vi "手动静音-网络版.vi"(9 "引用-通信单元-探头属性引用[]":refnum<vi>, 10 "引用-通信单元-改动项引用[]":refnum<vi>, 11 "引用-测量状态":refnum<vi>) -> ()   [LabVIEW 2017]
panel:
  in  "列表框":i32(listbox)
  out "映射-改动项引用[]":refnum<vi>[](array[refnum])
  in  "事件-选中行":refnum<user-event>
  in  "选中行":i32[](array[numeric])
  out "项数":i32
  out "信号-刷新列表":bool=TRUE
  in  "上翻":bool
  in  "全部静音":bool
  in  "下翻":bool
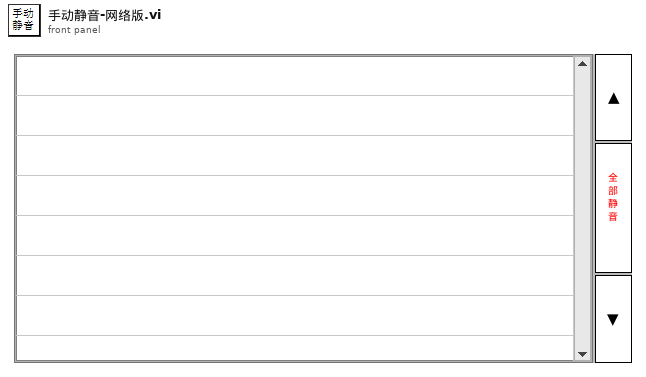
[diagram p1: front panel]
types:
  T1 = typedef "测量状态.ctl" = enum16{"正常", "一级报警", "二级报警", "累积报警", "有掉线"}
  T2 = typedef "改动项.ctl" = cluster{"改动项选择":T3, "启用？":bool, "探测器信息":T4}
  T3 = typedef "改动项选择.ctl" = enum16{"未改动", "改动-启用状态", "改动-探头信息", "改动-报警限值", "动作-手动静音", "动作-重启累积时段", "动作-累积删除", "动作-重连"}
  T4 = typedef "探测器信息.ctl" = cluster{"网络地址":string, "名称":string, "备注":string, "累积剂量":dbl, "累积限值":dbl, "硬件剂量率限值":T5, "剂量率限值1":dbl, "剂量率限值2":dbl, "报警方式":T6}
  T5 = typedef "探头剂量率限值选择.ctl" = enum16{"一级限值", "二级限值"}
  T6 = typedef "报警方式选择.ctl" = enum16{"常报警", "自动静音", "手动静音"}
  T7 = enum32{"Invalid", "Standard", "Closed", "Hidden", "Minimized", "Maximized"}
  T8 = typedef "探头属性.ctl" = cluster{"探头地址与信息":T4, "测量值":T9, "限值":T10, "探头状态":T11, "累积记录":T12, "报警方式":T13}
  T9 = typedef "测量值.ctl" = cluster{"时间":timestamp, "数值":dbl}
  T10 = typedef "剂量率限值.ctl" = cluster{"限值1":dbl, "限值2":dbl, "探头限值":T5}
  T11 = typedef "探头状态.ctl" = enum16{"正常", "离线", "禁用", "一级报警", "二级报警", "累积报警"}
  T12 = typedef "单条累积记录.ctl" = cluster{"起始时间":timestamp, "结束时间":timestamp, "累积剂量":dbl}
  T13 = typedef "报警方式.ctl" = cluster{"报警方式":T6, "延迟计时":u16, "报警中？":bool}
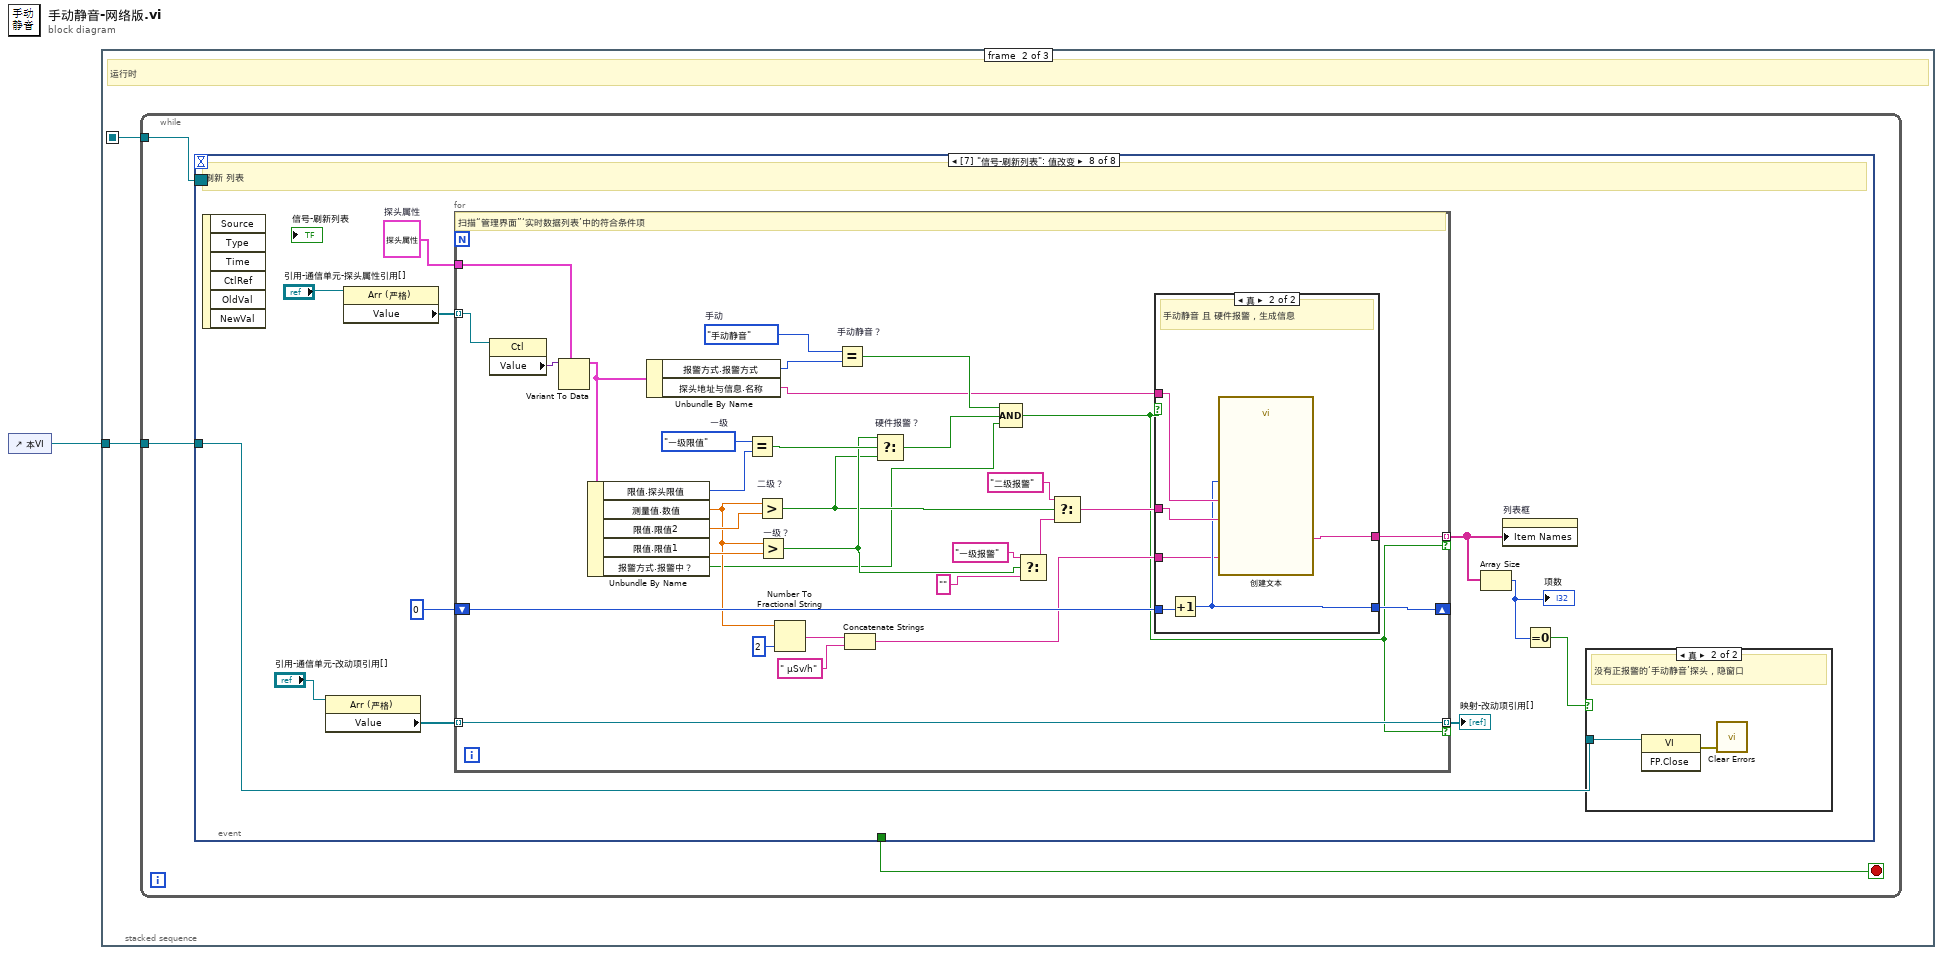
[diagram p0: block diagram]
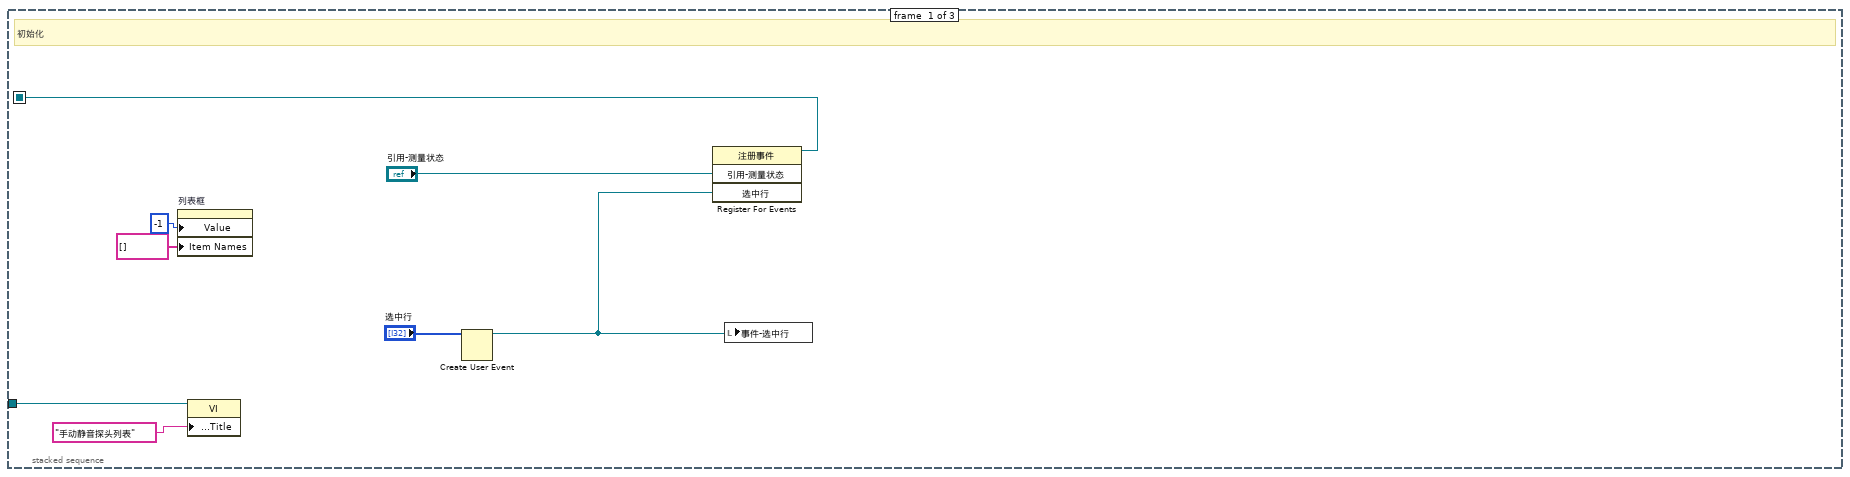
[diagram p2: hidden frame]
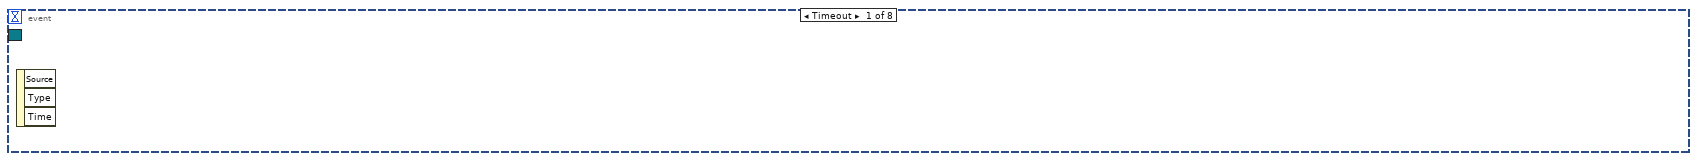
[diagram p3: hidden frame]
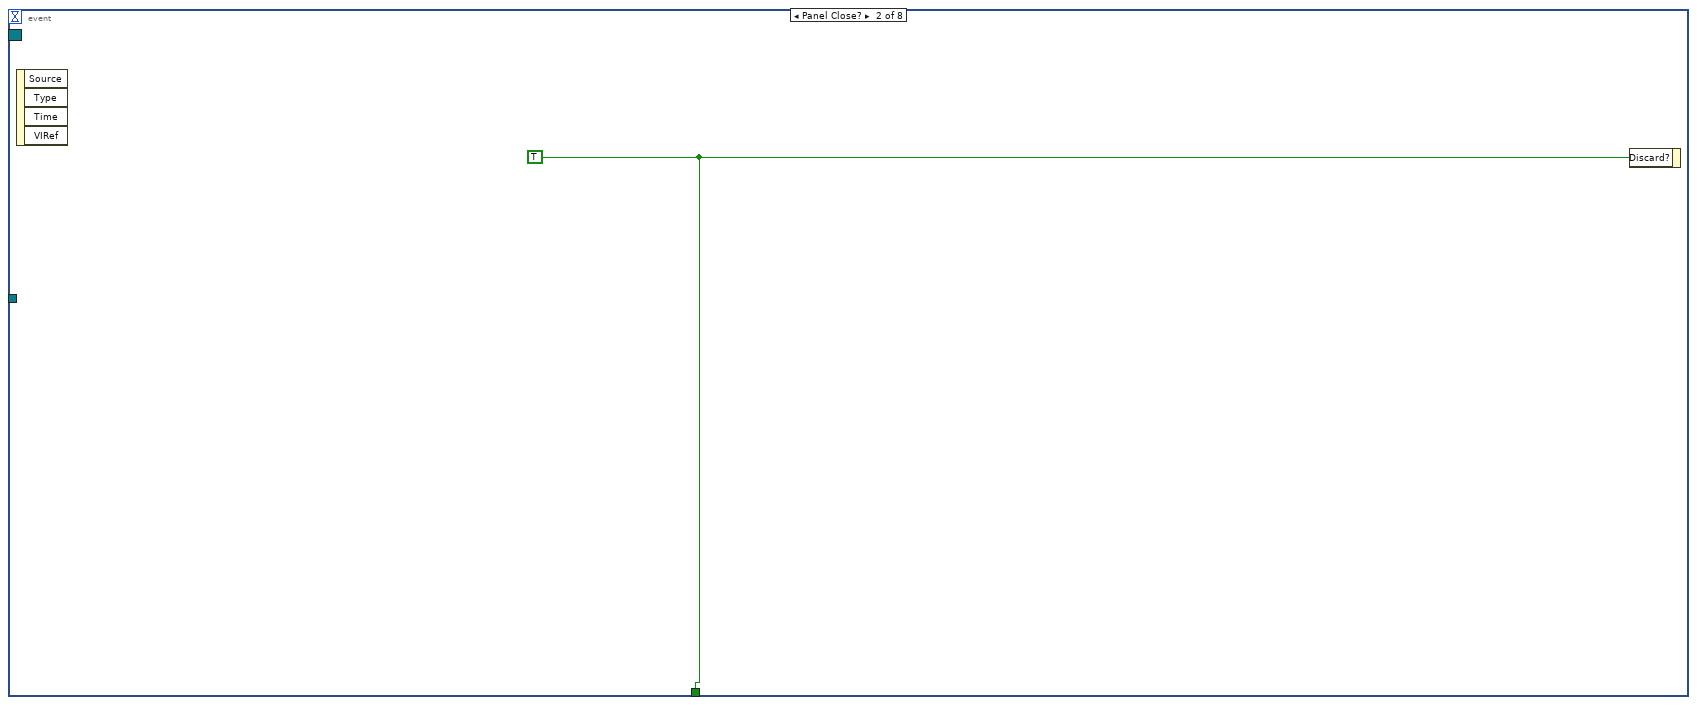
[diagram p4: hidden frame]
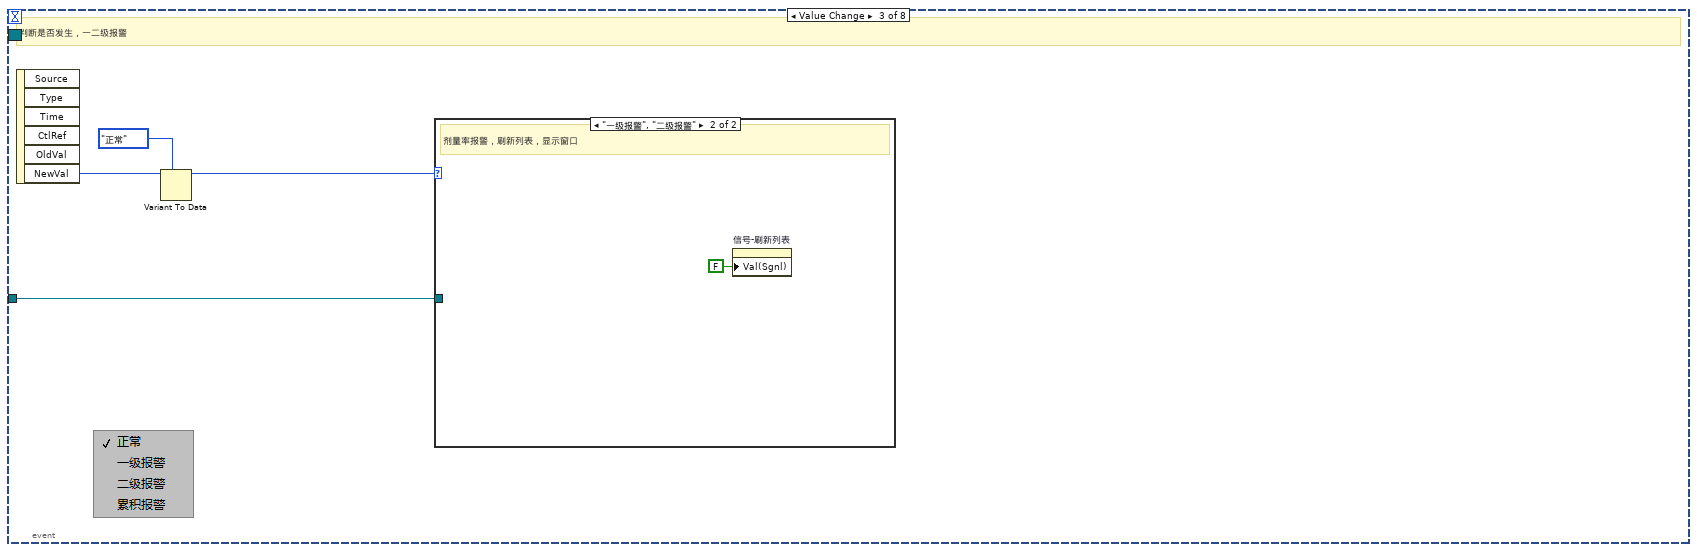
[diagram p5: hidden frame]
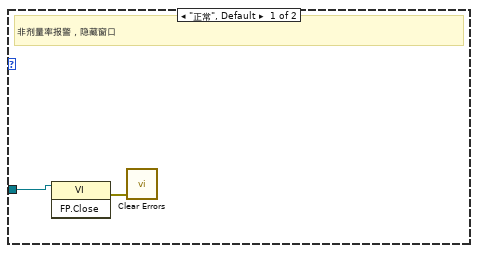
[diagram p6: hidden frame]
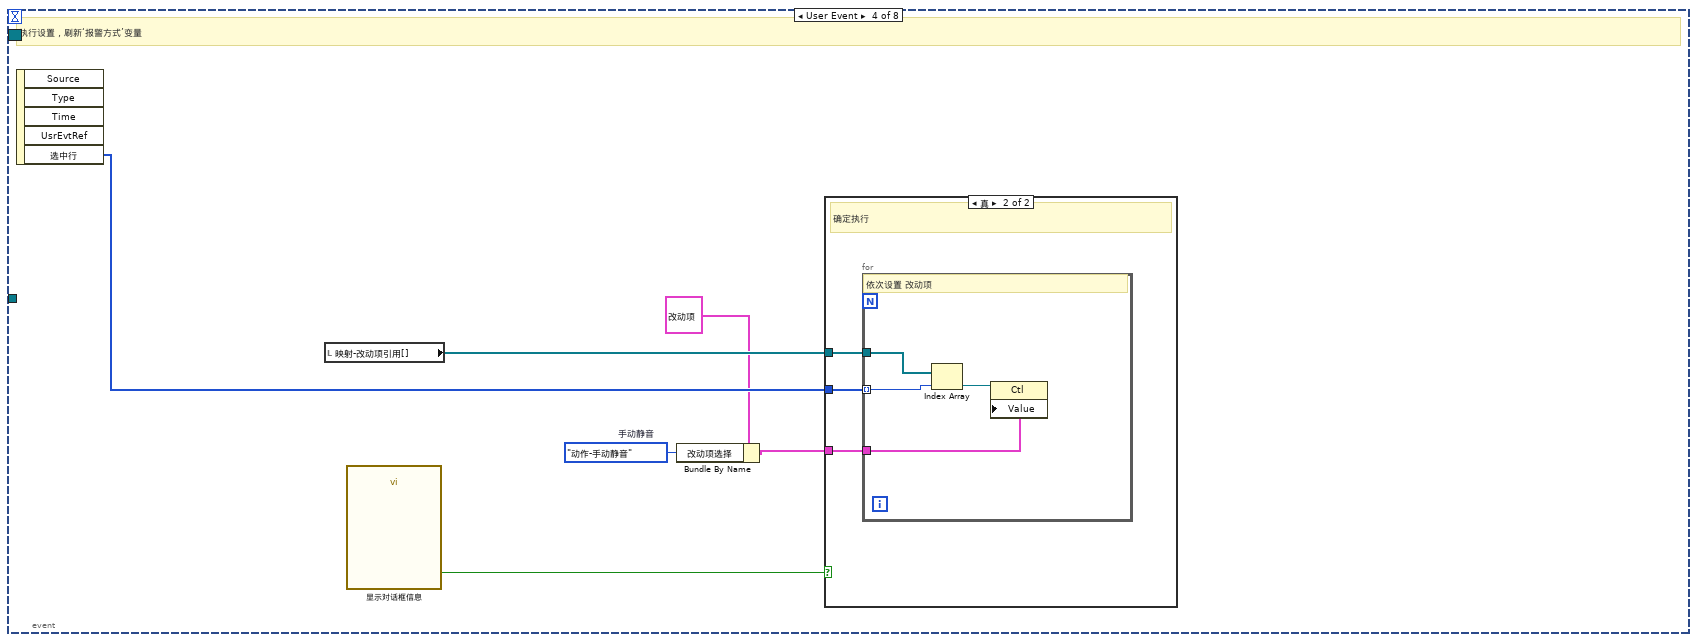
[diagram p7: hidden frame]
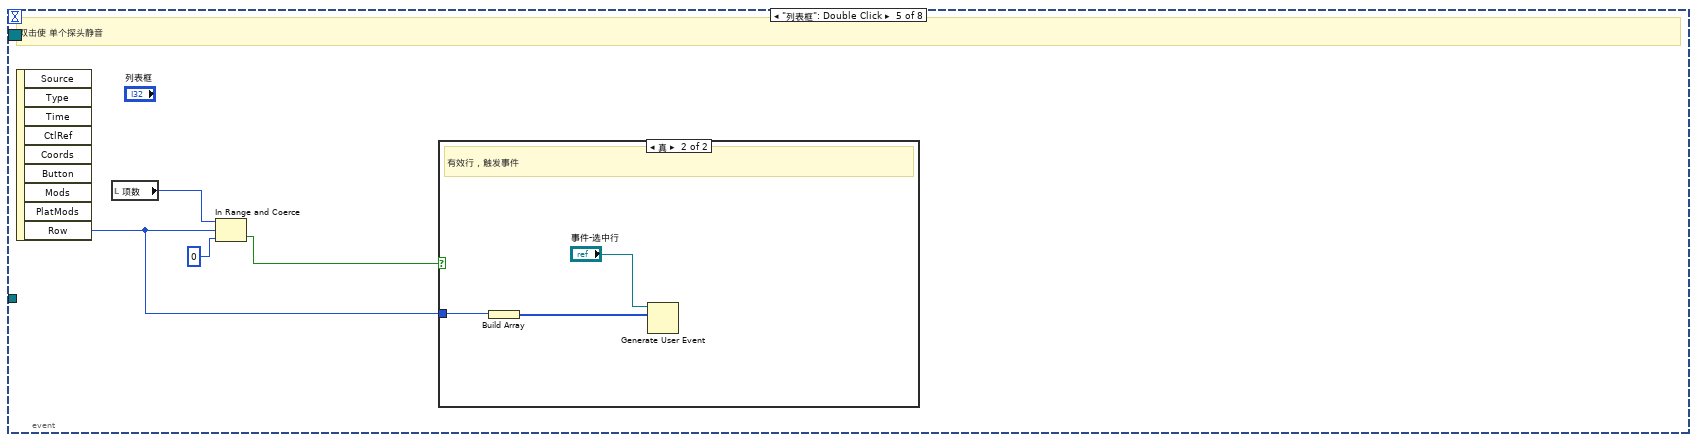
[diagram p9: hidden frame]
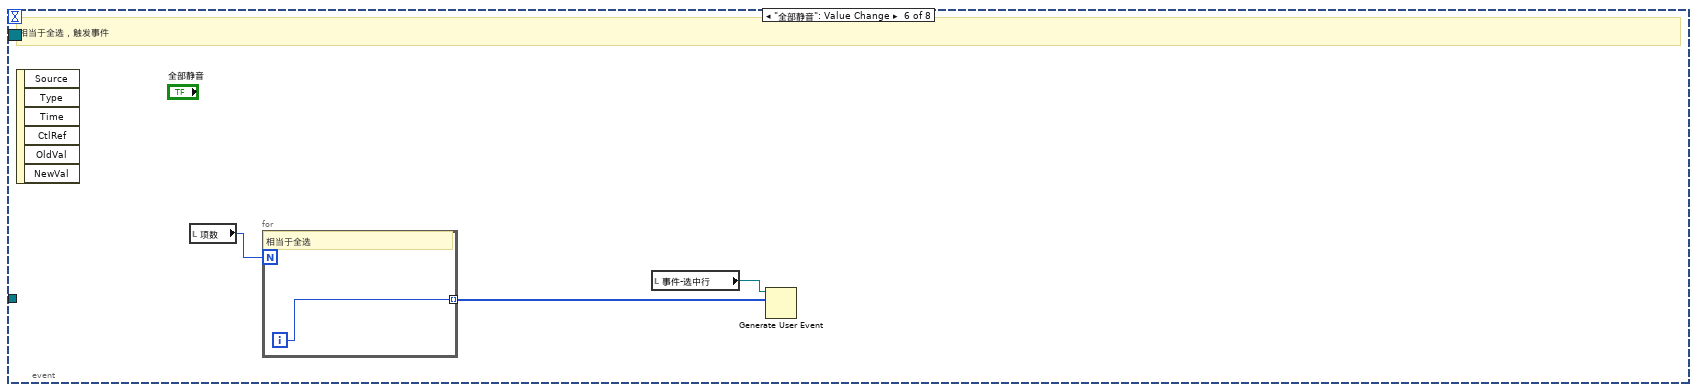
[diagram p11: hidden frame]
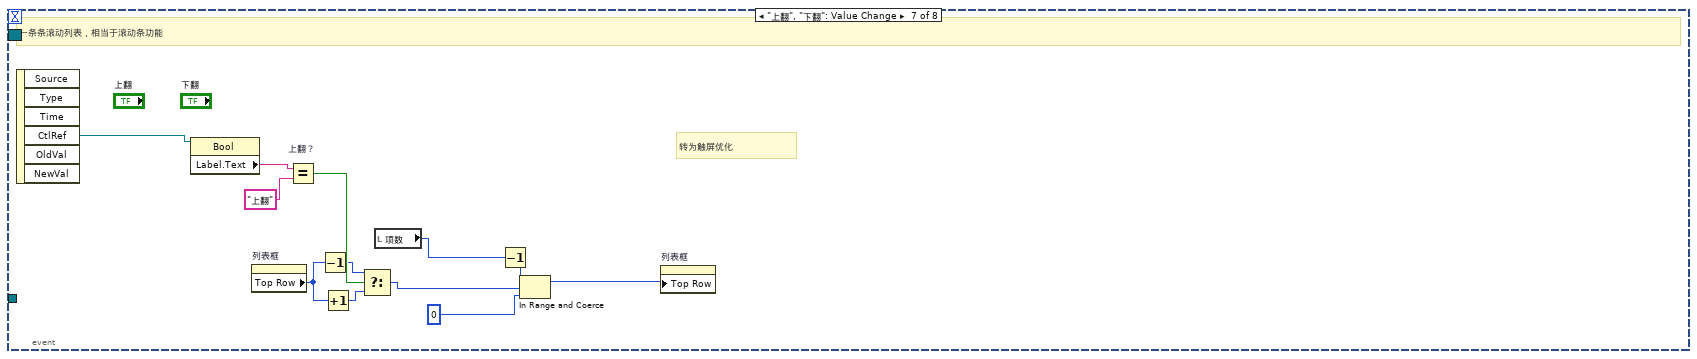
[diagram p12: hidden frame]
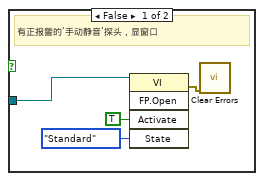
[diagram p13: hidden frame]
diagram:
  n1 = control-ref of="本VI"() -> (w1:refnum<vi>)
  n2 = stacked-sequence {
    seq-local: [w7 _ _] -> [_ w11 _]
    tunnel: w1 -> [w9 w10 _]
    frame #0 {
      # "初始化"
      n3 = property on="列表框" class="LstBox (严格)"("Value"=-1 ("列表框"), "Item Names"=string[] [] ("项名")) -> ()  [unwired: 2 in, 2 out]
      n4 = property class="VI"(reference=w9, "Front Panel.Title"="手动静音探头列表" ("前面板窗口:标题")) -> ()  [unwired: 1 in, 2 out]
      n5 = Create User Event(user event datatype="选中行") -> (user event=w3:refnum<user-event>)  [unwired: 1 in, 1 out]
      n6 = register-events("引用-测量状态", w3) -> (reference out=w7:refnum<event-registration>)  [unwired: 2 in, 1 out]
      n7 = local write "事件-选中行"(w3) -> ()
    }
    frame #1 {
      # "运行时"
      n8 = while {
        tunnel: w11 -> [w13]
        tunnel: w10 -> [w12]
        stop <- w14 stop-if-true
        n9 = event shown="[7] \"信号-刷新列表\": 值改变" {
          selector: w13 -> [_ _ _ _ _ _ _ _]
          dyn-events: _ -> [_ _ _ _ _ _ _ _]
          timeout: _ -> [_ _ _ _ _ _ _ _]
          tunnel: [_ w15 _ _ _ _ _ _] -> w14
          tunnel: w12 -> [_ _ w17 _ _ _ _ w66]
          event Timeout {
            n10 = event-data() -> ()  [unwired: 1 in, 3 out]
          }
          event Panel Close? {
            w15 = TRUE ("放弃？")
            n11 = event-data() -> ()  [unwired: 1 in, 4 out]
            n12 = event-data("Discard?"=w15) -> ()  [unwired: 1 in, 1 out]
          }
          event Value Change {
            # "判断是否发生，一二级报警"
            n13 = event-data() -> ("NewVal"=w18:T1)  [unwired: 1 in, 5 out]
            n14 = Variant To Data(type=测量状态."正常" ("测量状态"), Variant=w18) -> (data=w19:T1)  [unwired: 1 in, 1 out]
            n15 = case shown="\"一级报警\", \"二级报警\"" w19 {
              tunnel: w17 -> [w20 _]
              frame "正常", Default {
                # "非剂量率报警，隐藏窗口"
                n16 = invoke class="VI" method="FP.Close"(reference=w20) -> (error out=w21:errorcluster)  [unwired: 2 in, 2 out]
                n17 = call <vilib>:"Clear Errors.vi"("error in (no error)"=w21) -> ()  [unwired: 5 in, 2 out]
              }
              frame "一级报警", "二级报警" {
                # "剂量率报警，刷新列表，显示窗口"
                n18 = property on="信号-刷新列表" class="Bool (严格)"("Val(Sgnl)"=FALSE ("值(信号)")) -> ()  [unwired: 2 in, 2 out]
              }
            }
          }
          event User Event {
            w25 = 改动项选择."动作-手动静音"  # 手动静音
            # "执行设置，刷新‘报警方式’变量"
            n19 = event-data() -> ("选中行"=w28:i32[])  [unwired: 1 in, 4 out]
            n20 = local read "映射-改动项引用[]"() -> (w26:refnum<vi>[])
            n21 = call "显示对话框信息"() -> ("确定"=w27:bool)  [unwired: 10 in, 1 out]
            n22 = Bundle By Name(cluster=T2 {"改动项选择"=enum."未改动", "启用？"=FALSE, "探测器信息"={"网络地址"="", "名称"="", "备注"="", "累积剂量"=0.0, "累积限值"=0.0, "硬件剂量率限值"=enum."一级限值", "剂量率限值1"=0.0, "剂量率限值2"=0.0, "报警方式"=enum."常报警"}} ("改动项"), "改动项选择"=w25) -> (w23:T2)
            n23 = case shown="真" w27 {
              tunnel: w26 -> [_ w31]
              tunnel: w28 -> [_ w30]
              tunnel: w23 -> [_ w29]
              frame False {
                # "取消执行"
              }
              frame True {
                # "确定执行"
                n24 = for {
                  tunnel: w31 -> [w35]
                  tunnel: w30 -> [w34] mode=indexing
                  tunnel: w29 -> [w32]
                  # "依次设置 改动项"
                  n25 = Index Array(array=w35, index=w34) -> (element=w33:refnum<vi>)
                  n26 = property class="Ctl"(reference=w33, "Value"=w32) -> ()  [unwired: 1 in, 2 out]
                }
              }
            }
          }
          event "列表框": Double Click {
            # "双击使 单个探头静音"
            n27 = event-data() -> ("Row"=w36:i32)  [unwired: 1 in, 8 out]
            n28 = local read "项数"() -> (w38:i32)
            n29 = In Range and Coerce(upper limit=w38, x=w36, lower limit=0 ("下限")) -> (In Range?=w37:bool)  [unwired: 1 out]
            n30 = case shown="真" w37 {
              tunnel: w36 -> [_ w42]
              frame False {
                # "无效行"
              }
              frame True {
                # "有效行，触发事件"
                n31 = Build Array(w42) -> (w40:i32[])
                n32 = Generate User Event(user event="事件-选中行", event data cluster=w40) -> ()  [unwired: 2 in, 2 out]
              }
            }
          }
          event "全部静音": Value Change {
            # "相当于全选，触发事件"
            n33 = event-data() -> ()  [unwired: 1 in, 6 out]
            n34 = local read "项数"() -> (w45:i32)
            n35 = for {
              N: w45 -> [_]
              tunnel: [w46] -> w44 mode=indexing
              i -> [w46]
              # "相当于全选"
            }
            n36 = local read "事件-选中行"() -> (w43:refnum<user-event>)
            n37 = Generate User Event(user event=w43, event data cluster=w44) -> ()  [unwired: 2 in, 2 out]
          }
          event "上翻", "下翻": Value Change {
            # "转为触屏优化"
            # "一条条滚动列表，相当于滚动条功能"
            n38 = event-data() -> ("CtlRef"=w58:refnum<vi>)  [unwired: 1 in, 5 out]
            n39 = property class="Bool"(reference=w58) -> ("Label.Text"=w57:string)  [unwired: 1 in, 2 out]
            n40 = property on="列表框" class="LstBox (严格)"() -> ("Top Row"=w51:i32)  [unwired: 2 in, 2 out]
            n41 = Equal? "上翻？"(x=w57, y="上翻") -> (x = y?=w53:bool)
            n42 = Decrement(x=w51) -> (x-1=w52:i32)
            n43 = Increment(x=w51) -> (x+1=w50:i32)
            n44 = Select(t=w52, s=w53, f=w50) -> (s? t:f=w49:i32)
            n45 = local read "项数"() -> (w55:i32)
            n46 = Decrement(x=w55) -> (x-1=w47:i32)
            n47 = In Range and Coerce(upper limit=w47, x=w49, lower limit=0 ("下限")) -> (coerced(x)=w48:i32)  [unwired: 1 out]
            n48 = property on="列表框" class="LstBox (严格)"("Top Row"=w48) -> ()  [unwired: 2 in, 2 out]
          }
          event "信号-刷新列表": Value Change {
            w63 = T8 {"探头地址与信息"={"网络地址"="", "名称"="", "备注"="", "累积剂量"=0.0, "累积限值"=0.0, "硬件剂量率限值"=enum."一级限值", "剂量率限值1"=0.0, "剂量率限值2"=0.0, "报警方式"=enum."常报警"}, "测量值"={"时间"=timestamp(3554955153.6246996 s since 1904-01-01), "数值"=0.0}, "限值"={"限值1"=0.0, "限值2"=0.0, "探头限值"=enum."一级限值"}, "探头状态"=enum."正常", "累积记录"={"起始时间"=timestamp(0 s since 1904-01-01), "结束时间"=timestamp(0 s since 1904-01-01), "累积剂量"=0.0}, "报警方式"={"报警方式"=enum."常报警", "延迟计时"=0, "报警中？"=FALSE}}  # 探头属性
            # "刷新 列表"
            n49 = event-data() -> ()  [unwired: 1 in, 6 out]
            n50 = property class="Arr (严格)"(reference="引用-通信单元-改动项引用[]") -> ("Value"=w60:refnum<vi>[])  [unwired: 1 in, 2 out]
            n51 = property class="Arr (严格)"(reference="引用-通信单元-探头属性引用[]") -> ("Value"=w64:refnum<vi>[])  [unwired: 1 in, 2 out]
            n52 = for {
              tunnel: [w107] -> w69 mode=indexing if=w77
              tunnel: w64 -> [w106] mode=indexing
              tunnel: w63 -> [w104]
              shift-right: [w84] -> _
              shift-left: 0 -> [w85]
              tunnel: w60 -> [w78] mode=indexing
              tunnel: [w78] -> w59 mode=indexing if=w77
              w96 = 探头剂量率限值选择."一级限值"  # 一级
              w89 = 报警方式选择."手动静音"  # 手动
              # "扫描“管理界面”‘实时数据列表’中的符合条件项"
              n53 = property class="Ctl"(reference=w106) -> ("Value"=w105:variant)  [unwired: 1 in, 2 out]
              n54 = Variant To Data(type=w104, Variant=w105) -> (data=w91:T8)  [unwired: 1 in, 1 out]
              n55 = Unbundle By Name(w91) -> ("限值.探头限值"=w97:T5, "测量值.数值"=w82:dbl, "限值.限值2"=w103:dbl, "限值.限值1"=w102:dbl, "报警方式.报警中？"=w76:bool)
              n56 = Unbundle By Name(w91) -> ("报警方式.报警方式"=w90:T6, "探头地址与信息.名称"=w86:string)
              n57 = Equal?(x=w96, y=w97) -> (x = y?=w95:bool)
              n58 = Greater? "二级？"(x=w82, y=w103) -> (0:w93:bool)
              n59 = Greater? "一级？"(x=w82, y=w102) -> (0:w94:bool)
              n60 = Number To Fractional String(number=w82, precision (6)=i16 2 ("精度(6)")) -> (F-format string=w81:string)  [unwired: 2 in]
              n61 = Equal? "手动静音？"(x=w89, y=w90) -> (x = y?=w88:bool)
              n62 = Concatenate Strings(w81, " μSv/h" ("字符串")) -> (w79:string)
              n63 = Select "硬件报警？"(t=w94, s=w95, f=w93) -> (s? t:f=w92:bool)
              n64 = Compound Arithmetic op=AND ("复合运算")(w88, w92, w76) -> (w77:bool)
              n65 = Select(t="一级报警", s=w94, f="") -> (s? t:f=w98:string)
              n66 = Select(t="二级报警", s=w93, f=w98) -> (s? t:f=w87:string)
              n67 = case shown="真" w77 {
                tunnel: [_ w114] -> w107
                tunnel: w87 -> [_ w113]
                tunnel: w86 -> [_ w112]
                tunnel: w85 -> [w108 w111]
                tunnel: [w108 w110] -> w84
                tunnel: w79 -> [_ w109]
                frame False {
                  # "不符合条件"
                }
                frame True {
                  # "手动静音 且 硬件报警，生成信息"
                  n68 = Increment(x=w111) -> (x+1=w110:i32)
                  n69 = call "创建文本"("测量值"=w109, "序号"=w110, "探头名"=w112, "报警等级"=w113) -> ("Result"=w114:string)  [unwired: 10 in, 1 out]
                }
              }
            }
            "映射-改动项引用[]" <- w59
            n70 = Array Size(array=w69) -> (size(s)=w68:i32)
            "项数" <- w68
            n71 = property on="列表框" class="LstBox (严格)"("Item Names"=w69) -> ()  [unwired: 2 in, 2 out]
            n72 = Equal To 0?(x=w68) -> (x = 0?=w67:bool)
            n73 = case shown="真" w67 {
              tunnel: w66 -> [w70 w75]
              frame False {
                # "有正报警的‘手动静音’探头，显窗口"
                n74 = invoke class="VI" method="FP.Open"(reference=w70, "Activate"=TRUE ("激活？"), "State"=T7."Standard" ("状态")) -> (error out=w71:errorcluster)  [unwired: 2 in, 4 out]
                n75 = call <vilib>:"Clear Errors.vi"("error in (no error)"=w71) -> ()  [unwired: 5 in, 2 out]
              }
              frame True {
                # "没有正报警的‘手动静音’探头，隐窗口"
                n76 = invoke class="VI" method="FP.Close"(reference=w75) -> (error out=w74:errorcluster)  [unwired: 2 in, 2 out]
                n77 = call <vilib>:"Clear Errors.vi"("error in (no error)"=w74) -> ()  [unwired: 5 in, 2 out]
              }
            }
          }
        }
      }
    }
    frame #2 {
      # "结束"
    }
  }
